vi "ZeroStage.vi"(11 "milliseconds to wait":u32) -> ()   [LabVIEW 2020]
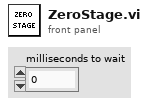
[diagram p1: front panel]
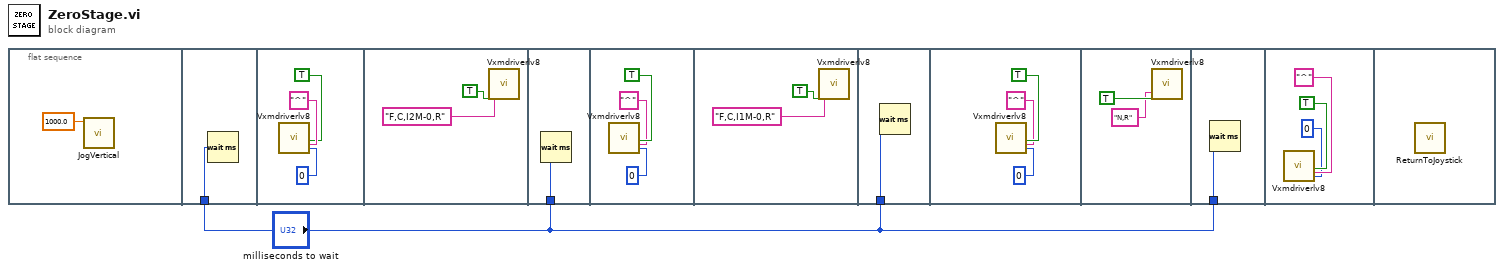
[diagram p0: block diagram]
diagram:
  n1 = flat-sequence {
    tunnel: "milliseconds to wait" -> [w3]
    tunnel: "milliseconds to wait" -> [w9]
    tunnel: "milliseconds to wait" -> [w15]
    tunnel: "milliseconds to wait" -> [w21]
    frame #0 {
      n2 = call "JogVertical.vi"("Numeric"=1000.0) -> ()  [unwired: 11 in]
    }
    frame #1 {
      n3 = Wait (ms)(milliseconds to wait=w3) -> ()  [unwired: 1 out]
    }
    frame #2 {
      n4 = call "Vxmdriverlv8.Vi"("Wait\nfor \nchar"=TRUE, "Char(s) to wait for"="^", "Char\nTimeout\nTime (ms)"=0) -> ()  [unwired: 19 in, 6 out]
    }
    frame #3 {
      n5 = call "Vxmdriverlv8.Vi"("Send\nchars\nto port"=TRUE, "Chars to send"="F,C,I2M-0,R") -> ()  [unwired: 20 in, 6 out]
    }
    frame #4 {
      n6 = Wait (ms)(milliseconds to wait=w9) -> ()  [unwired: 1 out]
    }
    frame #5 {
      n7 = call "Vxmdriverlv8.Vi"("Wait\nfor \nchar"=TRUE, "Char(s) to wait for"="^", "Char\nTimeout\nTime (ms)"=0) -> ()  [unwired: 19 in, 6 out]
    }
    frame #6 {
      n8 = call "Vxmdriverlv8.Vi"("Send\nchars\nto port"=TRUE, "Chars to send"="F,C,I1M-0,R") -> ()  [unwired: 20 in, 6 out]
    }
    frame #7 {
      n9 = Wait (ms)(milliseconds to wait=w15) -> ()  [unwired: 1 out]
    }
    frame #8 {
      n10 = call "Vxmdriverlv8.Vi"("Wait\nfor \nchar"=TRUE, "Char(s) to wait for"="^", "Char\nTimeout\nTime (ms)"=0) -> ()  [unwired: 19 in, 6 out]
    }
    frame #9 {
      n11 = call "Vxmdriverlv8.Vi"("Send\nchars\nto port"=TRUE, "Chars to send"="N,R") -> ()  [unwired: 20 in, 6 out]
    }
    frame #10 {
      n12 = Wait (ms)(milliseconds to wait=w21) -> ()  [unwired: 1 out]
    }
    frame #11 {
      n13 = call "Vxmdriverlv8.Vi"("Wait\nfor \nchar"=TRUE, "Char(s) to wait for"="^", "Char\nTimeout\nTime (ms)"=0) -> ()  [unwired: 19 in, 6 out]
    }
    frame #12 {
      n14 = call "ReturnToJoystick.vi"() -> ()  [unwired: 12 in]
    }
  }
